vi "StringToBase64_NiVerified.vi"(8 "error in":errorcluster, 10 "Encode":bool, 11 "RawString":string) -> (0 "error out":errorcluster, 3 "EncodedString":string)   [LabVIEW 2024, in "OpenLvVision_Image.lvlib" / "File.lvlib"]
doc: "Converts a string to uri base 64 encoded string"
uses:
  File.lvlib
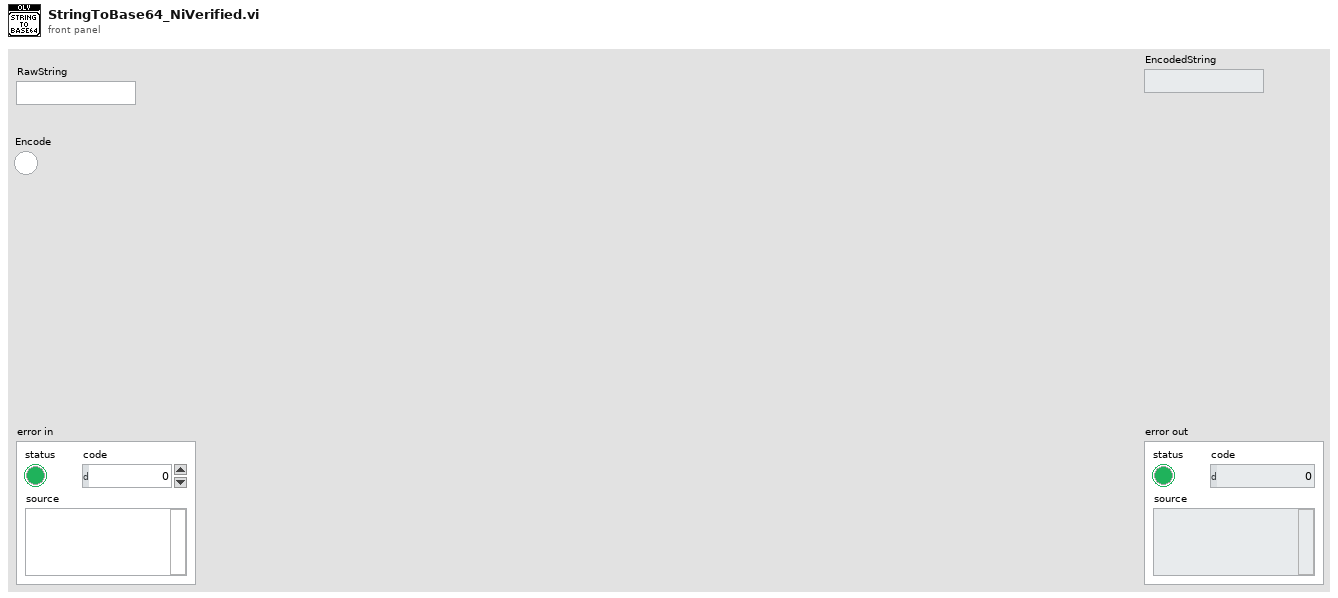
[diagram p1: front panel]
types:
  T1 = cluster{"unsigned byte array[0]":u8, "unsigned byte array[1]":u8, "unsigned byte array[2]":u8}
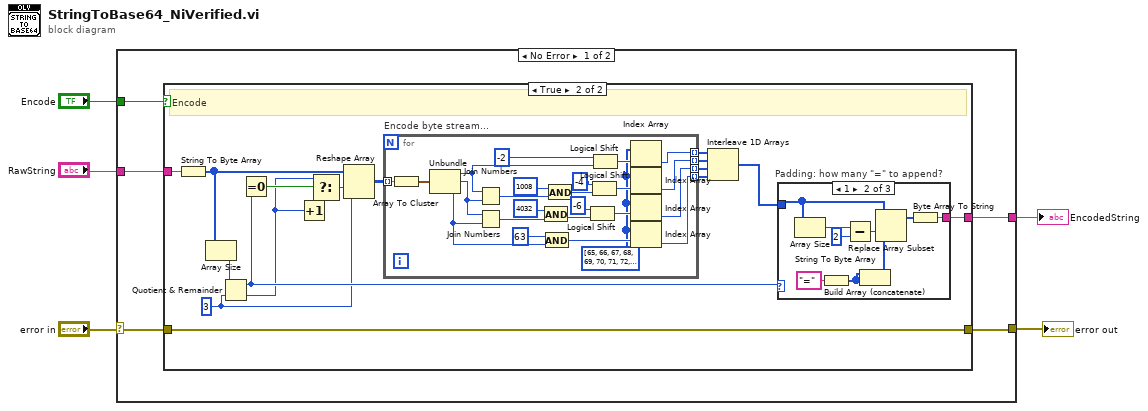
[diagram p0: block diagram]
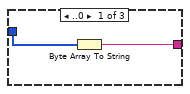
[diagram p3: hidden frame]
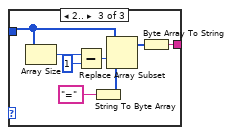
[diagram p4: hidden frame]
diagram:
  n1 = case shown="No Error" "error in" {
    selector: "error in" -> [w6 w74]
    tunnel: "RawString" -> [w10 w73]
    tunnel: [w7 w74] -> w4
    tunnel: [w9 w73] -> w3
    tunnel: "Encode" -> [w8 _]
    frame No Error {
      n2 = case shown="True" w8 {
        tunnel: w10 -> [w12 w16]
        tunnel: [w12 w15] -> w9
        tunnel: [w11 w13] -> w7
        tunnel: w6 -> [w11 w13]
        frame False {
        }
        frame True {
          w19 = 3 ("y")
          # "Encode"
          n3 = String To Byte Array(string=w16) -> (unsigned byte array=w20:u8[])
          n4 = Array Size(array=w20) -> (size(s)=w27:i32)
          n5 = Quotient & Remainder(x=w27, y=w19) -> (x-y*floor(x/y)=w28:i32, floor(x/y)=w21:i32)
          n6 = Equal To 0?(x=w28) -> (x = 0?=w29:bool)
          n7 = Increment(x=w21) -> (x+1=w22:i32)
          n8 = Select(t=w21, s=w29, f=w22) -> (s? t:f=w18:i32)
          n9 = Reshape Array(w20, w18, w19) -> (w17:u8[][])
          n10 = for "Encode byte stream..." {
            tunnel: [w32] -> w23 mode=indexing
            tunnel: [w33] -> w24 mode=indexing
            tunnel: [w34] -> w25 mode=indexing
            tunnel: [w35] -> w26 mode=indexing
            tunnel: w17 -> [w30] mode=indexing
            w31 = u8[] [65, 66, 67, 68, 69, 70, 71, 72, 73, 74, 75, 76, 77, 78, 79, 80, 81, 82, 83, 84, 85, 86, 87, 88, 89, 90, 97, 98, 99, 100, 101, 102, 103, 104, 105, 106, 107, 108, 109, 110, 111, 112, 113, 114, 115, 116, 117, 118, 119, 120, 121, 122, 48, 49, 50, 51, 52, 53, 54, 55, 56, 57, 43, 47] ("unsigned byte array")
            n11 = Array To Cluster(array=w30) -> (cluster=w53:T1)
            n12 = Unbundle(w53) -> ("unsigned byte array[0]"=w42:u8, "unsigned byte array[1]"=w47:u8, "unsigned byte array[2]"=w41:u8)
            n13 = Join Numbers(hi=w42, lo=w47) -> ((hi.lo)=w51:u16)
            n14 = Join Numbers(hi=w47, lo=w41) -> ((hi.lo)=w46:u16)
            n15 = And(x=u16 4032, y=w46) -> (x .and. y?=w44:u16)
            n16 = And(x=u8 63, y=w41) -> (x .and. y?=w36:u8)
            n17 = And(x=u16 1008, y=w51) -> (x .and. y?=w49:u16)
            n18 = Logical Shift(y=i8 -6, x=w44) -> (x << y=w37:u16)
            n19 = Logical Shift(y=i8 -4, x=w49) -> (x << y=w38:u16)
            n20 = Logical Shift(y=i8 -2, x=w42) -> (x << y=w39:u8)
            n21 = Index Array(array=w31, index=w39) -> (element=w35:u8)
            n22 = Index Array(array=w31, index=w38) -> (element=w34:u8)
            n23 = Index Array(array=w31, index=w37) -> (element=w33:u8)
            n24 = Index Array(array=w31, index=w36) -> (element=w32:u8)
          }
          n25 = Interleave 1D Arrays(w26, w25, w24, w23) -> (w14:u8[])
          n26 = case "Padding: how many \"=\" to append?" shown="1" w28 {
            tunnel: [w54 w61 w69] -> w15
            tunnel: w14 -> [w55 w59 w67]
            frame ..0 {
              n27 = Byte Array To String(unsigned byte array=w55) -> (string=w54:string)
            }
            frame 1 {
              n28 = Array Size(array=w59) -> (size(s)=w60:i32)
              n29 = String To Byte Array(string="=") -> (unsigned byte array=w57:u8[])
              n30 = Subtract(x=w60, y=2) -> (x-y=w63:i32)
              n31 = Build Array (concatenate)(w57, w57) -> (w56:u8[])
              n32 = Replace Array Subset(array=w59, new element=w56, index=w63) -> (w62:u8[])
              n33 = Byte Array To String(unsigned byte array=w62) -> (string=w61:string)
            }
            frame 2.. {
              n34 = Array Size(array=w67) -> (size(s)=w68:i32)
              n35 = Subtract(x=w68, y=1) -> (x-y=w71:i32)
              n36 = String To Byte Array(string="=") -> (unsigned byte array=w65:u8[])
              n37 = Replace Array Subset(array=w67, new element=w65, index=w71) -> (w70:u8[])
              n38 = Byte Array To String(unsigned byte array=w70) -> (string=w69:string)
            }
          }
        }
      }
    }
    frame Error {
    }
  }
  "error out" <- w4
  "EncodedString" <- w3
